vi "NX Initial Command.vi"(2 "z offset":dbl, 3 "x offset":dbl, 4 "y offset":dbl, 5 "selected path":path) -> (1 "3D comet":refnum<class "3D Plot Datatype.lvclass">[](array[class]))   [LabVIEW 2015]
uses:
  <vilib>/Math Plots/3D Math Plots/3D Plot/3D Plot Datatype/3D Plot Datatype.lvclass
  <vilib>/Math Plots/3D Math Plots/3D Comet/3D Comet XCtrl/3D Comet.xctl
  Globals.vi
  <vilib>/Math Plots/3D Math Plots/3D Comet/3D Comet Datatype/Public/Plot Helper (Vector).vi
  <vilib>/Math Plots/3D Math Plots/3D Comet/3D Comet Datatype/3D Comet Datatype.lvclass
panel:
  out "deleted portion":dbl[](array[numeric])
  out "3D Comet":refnum<class "3D Plot Datatype.lvclass">[](xcontrol)
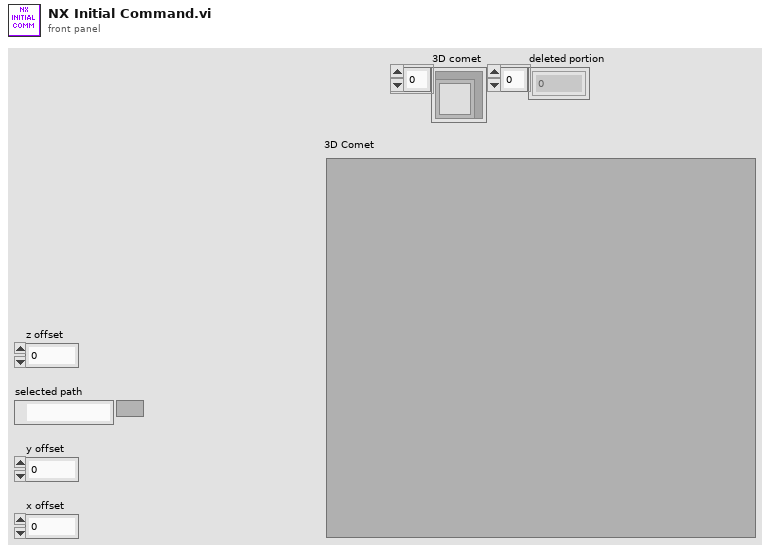
[diagram p1: front panel]
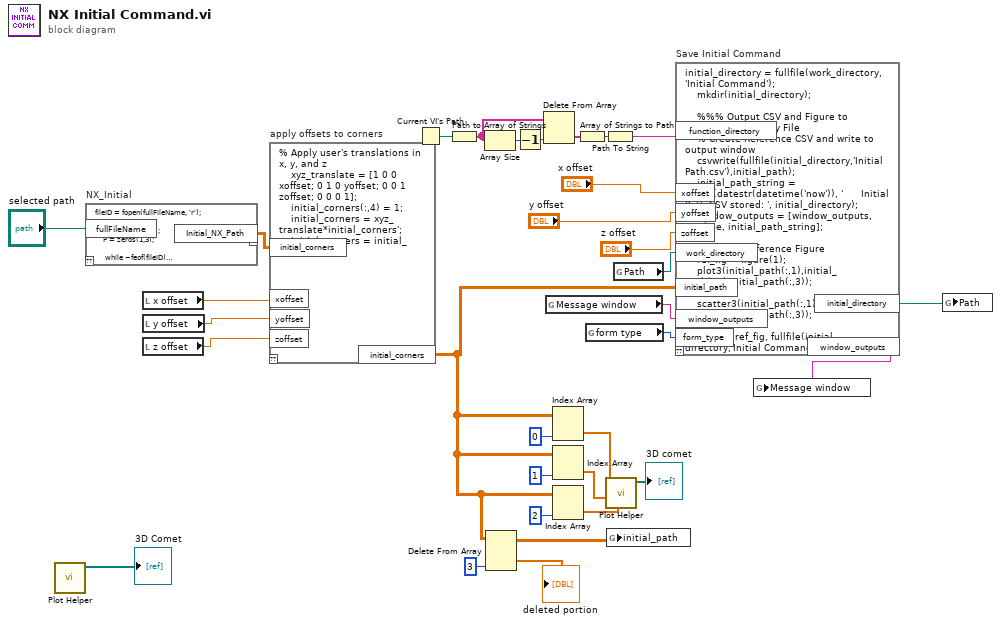
[diagram p0: block diagram]
diagram:
  n1 = call-poly <vilib>:"Plot Helper.vi"() -> ("3D Plot lvclass Array out"=→"3D Comet":refnum<class "3D Plot Datatype.lvclass">[])  [unwired: 6 in, 5 out]
  n2 = script code="fileID = fopen(fullFileName, 'r');\n\n    index = int64(1);\n    P = zeros(1,3);\n\n     while ~feof(fileID)\n        templine = fgetl(fileID);\n        if strcmp(templine, \"\") %if empty, skip\n            %nothing\n        else %if line starts with GOTO/\n            if strcmp(templine(1:1), 'G')\n                Pstring{index, 1} = templine;\n                contents = Pstring{index};\n                Pstring{index} = contents(6:end);%trim off GOTO/ from line\n                Temp = str2num(Pstring{index});\n                Initial_NX_Path(index, 1) = Temp(1); %x\n                Initial_NX_Path(index, 2) = Temp(2); %y\n                Initial_NX_Path(index, 3) = Temp(3); %z\n                index = index + 1; \n            end\n        end\n     end\n \n\n    fclose(fileID);\n\n    \n    plot3(Initial_NX_Path(:,1),Initial_NX_Path(:,2),Initial_NX_Path(:,3),'k');\n    hold on;\n    scatter3(Initial_NX_Path(:,1),Initial_NX_Path(:,2),Initial_NX_Path(:,3),'b');\n    hold off;\n   \n    xlabel(\"X (mm)\");\n    ylabel(\"Y (mm)\");\n    zlabel(\"Z (mm)\");" "NX_Initial"("fullFileName"="selected path") -> ("Initial_NX_Path"=w17:dbl[][])  [unwired: 1 in, 1 out]
  n3 = local read "x offset"() -> (w13:dbl)
  n4 = local read "y offset"() -> (w14:dbl)
  n5 = local read "z offset"() -> (w15:dbl)
  n6 = script code="% Apply user's translations in x, y, and z\n    xyz_translate = [1 0 0 xoffset; 0 1 0 yoffset; 0 0 1 zoffset; 0 0 0 1];\n    initial_corners(:,4) = 1;\n    initial_corners = xyz_translate*initial_corners';\n    initial_corners = initial_corners';" "apply offsets to corners"("initial_corners"=w17, "yoffset"=w14, "zoffset"=w15, "xoffset"=w13) -> ("initial_corners"=w4:dbl[][])  [unwired: 1 in, 1 out]
  n7 = Current VI's Path() -> (path=w20:path)
  n8 = Path to Array of Strings(0:w20) -> (2:w19:string[])  [unwired: 1 out]
  n9 = Array Size(array=w19) -> (size(s)=w22:i32)
  n10 = Delete From Array(array=w4, index (col)=3 ("disabled index (col)")) -> (deleted portion=→"deleted portion":dbl[], array with subset deleted=w1:dbl[][])  [unwired: 2 in]
  n11 = Decrement(x=w22) -> (x-1=w23:i32)
  n12 = Delete From Array(array=w19, index=w23) -> (array with subset deleted=w21:string[])  [unwired: 1 in, 1 out]
  n13 = global read "Globals.vi" "Message window"() -> (w26:string)
  n14 = Index Array(array=w4, index (col)=0 ("disabled index (col)")) -> (element=w12:dbl[])  [unwired: 1 in]
  n15 = Index Array(array=w4, index (col)=1 ("disabled index (col)")) -> (element=w11:dbl[])  [unwired: 1 in]
  n16 = Index Array(array=w4, index (col)=2 ("disabled index (col)")) -> (element=w10:dbl[])  [unwired: 1 in]
  n17 = Array of Strings to Path(0:w21) -> (2:w24:path)  [unwired: 1 in]
  n18 = global read "Globals.vi" "form type"() -> (w25:u16)
  n19 = Path To String(path=w24) -> (string=w18:string)
  n20 = call-poly <vilib>:"Plot Helper.vi"("z vector"=w10, "y vector"=w11, "x vector"=w12) -> ("3D Plot lvclass Array out"=→"3D comet":refnum<class "3D Plot Datatype.lvclass">[])  [unwired: 3 in, 5 out]
  n21 = global write "Globals.vi" "initial_path"(w1) -> ()
  n22 = global read "Globals.vi" "Path"() -> (w30:path)
  n23 = script code="initial_directory = fullfile(work_directory, 'Initial Command');\n    mkdir(initial_directory);\n\n    %%% Output CSV and Figure to Reference Directory File\n    % Create Reference CSV and write to output window\n    csvwrite(fullfile(initial_directory,'Initial Path.csv'),initial_path);\n    initial_path_string = strcat(datestr(datetime('now')), '      Initial Path CSV stored: ', initial_directory);\n    window_outputs = [window_outputs, newline, initial_path_string];   \n\n    % Create Reference Figure    \n    ref_fig = figure(1);\n    plot3(initial_path(:,1),initial_path(:,2),initial_path(:,3));\n    hold on\n    scatter3(initial_path(:,1),initial_path(:,2),initial_path(:,3));\n    hold off\n    savefig(ref_fig, fullfile(initial_directory,'Initial Command Figure.fig'));\n\n    initial_fig_string = strcat(datestr(datetime('now')), '      Initial Figure stored:  ', initial_directory);\n    window_outputs = [window_outputs, newline, initial_fig_string];\n    \n    %%% Create command for robot based on initial_path\n    oldDir = pwd;\n    cd(function_directory)\n    Module_Output(initial_path, initial_directory);\n    cd(oldDir);\n\n    module_string = strcat(datestr(datetime('now')), '      Initial Module file stored:  ', initial_directory);\n    window_outputs = [window_outputs, newline, module_string];\n\n    % Print line divider to output window\n    window_outputs = [window_outputs, newline, ' ----------- ', newline];\n    \n\n        %%% Save inputs to work space\n        fileID = fopen(fullfile(initial_directory,'Initial Pyramid Parameters.txt'),'w');\n        fprintf(fileID,'Initial Parameters\\n');\n        fprintf(fileID,'X offset (mm): %4.3f\\n',xoffset);\n        fprintf(fileID,'Y offset (mm): %4.3f\\n',yoffset);\n        fprintf(fileID,'Z offset (mm): %4.3f\\n',zoffset);\n        fclose(fileID);" "Save Initial Command"("work_directory"=w30, "initial_path"=w4, "window_outputs"=w26, "form_type"=w25, "xoffset"="x offset", "yoffset"="y offset", "zoffset"="z offset", "function_directory"=w18) -> ("initial_directory"=w32:path, "window_outputs"=w31:string)  [unwired: 1 in, 1 out]
  n24 = global write "Globals.vi" "Message window"(w31) -> ()
  n25 = global write "Globals.vi" "Path"(w32) -> ()
